vi "1.1.vi"(9 "n":u32) -> (1 "fib(n)":i32)   [LabVIEW 2013]
panel:
  out "Array":i32[](array[numeric])
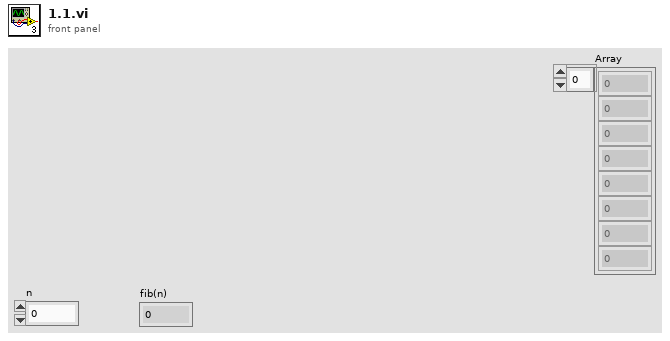
[diagram p1: front panel]
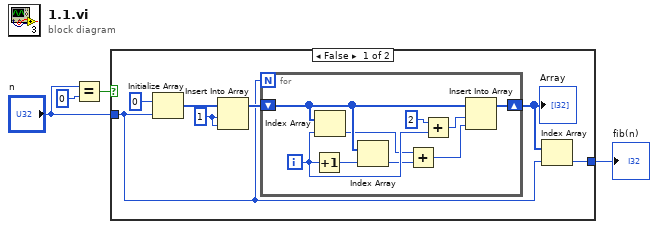
[diagram p0: block diagram]
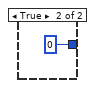
[diagram p2: hidden frame]
diagram:
  n1 = Equal?(x="n", y=u32 0) -> (x = y?=w1:bool)
  n2 = case shown="False" w1 {
    tunnel: "n" -> [w6 _]
    tunnel: [w5 0] -> w2
    frame False {
      w9 = 1 ("index")
      n3 = Initialize Array(0 ("element"), w6) -> (w10:i32[])
      n4 = Insert Into Array(array=w10, index=w9, new element=w9) -> (w8:i32[])
      n5 = for {
        N: w6 -> [_]
        shift-right: [w20] -> w7
        shift-left: w8 -> [w17]
        i -> [w16]
        n6 = Increment(x=w16) -> (x+1=w15:i32)
        n7 = Index Array(array=w17, index=w16) -> (element=w14:i32)
        n8 = Index Array(array=w17, index=w15) -> (element=w13:i32)
        n9 = Add(x=w14, y=w13) -> (x+y=w12:i32)
        n10 = Add(x=2, y=w16) -> (x+y=w18:i32)
        n11 = Insert Into Array(array=w17, index=w18, new element=w12) -> (w20:i32[])
      }
      "Array" <- w7
      n12 = Index Array(array=w7, index=w6) -> (element=w5:i32)
    }
    frame True {
    }
  }
  "fib(n)" <- w2
